vi "Stop.vi"(8 "error in (no error)":errorcluster, 11 "ArrayManager in":refnum<class "ArrayManager.lvclass">) -> (0 "error out":errorcluster, 3 "ArrayManager out":refnum<class "ArrayManager.lvclass">)   [LabVIEW 2014, in "OOPanel.lvlib" / "ArrayManager.lvclass"]
uses:
  ArrayManager.lvclass
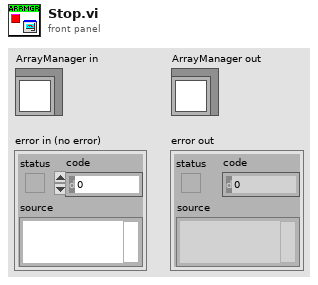
[diagram p1: front panel]
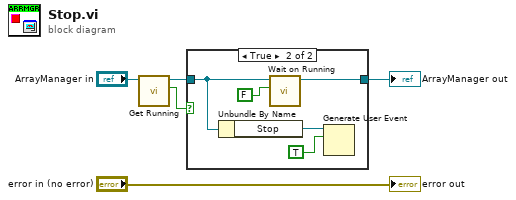
[diagram p0: block diagram]
diagram:
  n1 = call "Get Running.vi"("ArrayManager in"="ArrayManager in") -> ("Running"=w1:bool, "ArrayManager out"=w3:refnum<class "ArrayManager.lvclass">)  [unwired: 8 in, 1 out]
  n2 = case shown="True" w1 {
    tunnel: w3 -> [w6 w9]
    tunnel: [w6 w8] -> w2
    frame False {
    }
    frame True {
      n3 = Unbundle By Name(w9) -> ("Stop"=w11:refnum<user-event>)
      n4 = call "Wait on Running.vi"("Value"=FALSE, "ArrayManager in"=w9) -> ("ArrayManager out"=w8:refnum<class "ArrayManager.lvclass">)  [unwired: 8 in, 1 out]
      n5 = Generate User Event(user event=w11, event data cluster=TRUE ("event data")) -> ()  [unwired: 2 in, 2 out]
    }
  }
  "ArrayManager out" <- w2
  "error out" <- "error in (no error)"
